vi "Get Variant.vi"(8 "error in (no error)":errorcluster, 11 "VariantMsg In":refnum<class "VariantMsg.lvclass">) -> (0 "error out":errorcluster, 2 "Message Data":variant, 3 "VariantMsg Out":refnum<class "VariantMsg.lvclass">)   [LabVIEW 2018, in "LapDog.Messaging.v3.NativeTypes.lvlib" / "VariantMsg.lvclass"]
doc: "Returns the data contained in the message.\n\nThis method executes regardless of the error in state."
uses:
  VariantMsg.lvclass
  VariantMsg.lvclass/VariantMsg.ctl
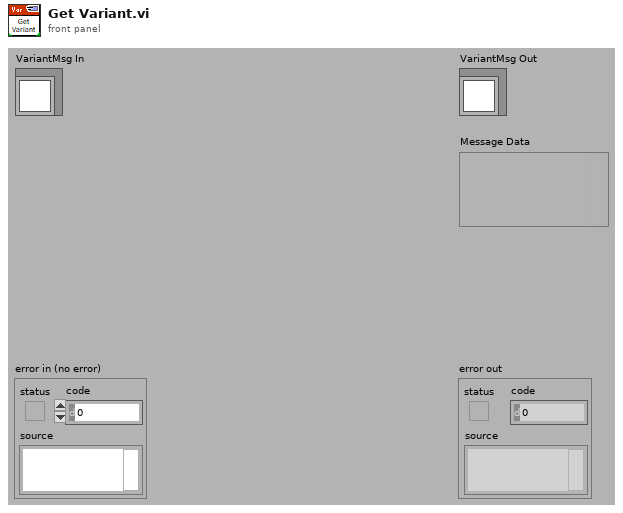
[diagram p1: front panel]
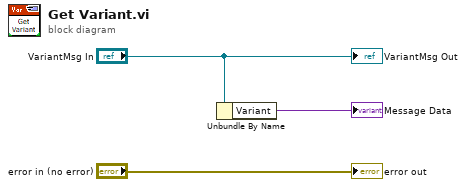
[diagram p0: block diagram]
diagram:
  n1 = Unbundle By Name("VariantMsg In") -> ("Variant"=→"Message Data":variant)
  "error out" <- "error in (no error)"
  "VariantMsg Out" <- "VariantMsg In"
